vi "ACal-Create Cal Sweep.vi"(8 "error in (no error)":errorcluster, 11 "Cal Stimulus":T1={"Min Freq (Hz)"=50.0, "Max Freq (Hz)"=50000.0, "Freq Step (Hz)"=50.0, "Waveform"=enum."Chirp", "Attenuation (dB)"=20.0, "Sample Rate (Hz)"=100000.0}) -> (0 "error out":errorcluster, 2 "Stimulus waveform":cluster{i32, dbl, dbl[]}, 3 "Stimulus":dbl[](array[numeric]))   [LabVIEW 2020]
uses:
  Type Defs/Cal Stimulus.ctl
  <vilib>/Analysis/2dsp.llb/Inverse Complex FFT.vi
  <vilib>/Analysis/NI_AALPro.lvlib
panel:
  out "Phase graph":cluster{i32, "Freq Step (Hz)":dbl, dbl[]}(graph)
  out "Magnitude graph":cluster{i32, "Freq Step (Hz)":dbl, dbl[]}(graph)
  out "Signal graph":cluster{i32, dbl, dbl[]}(graph)
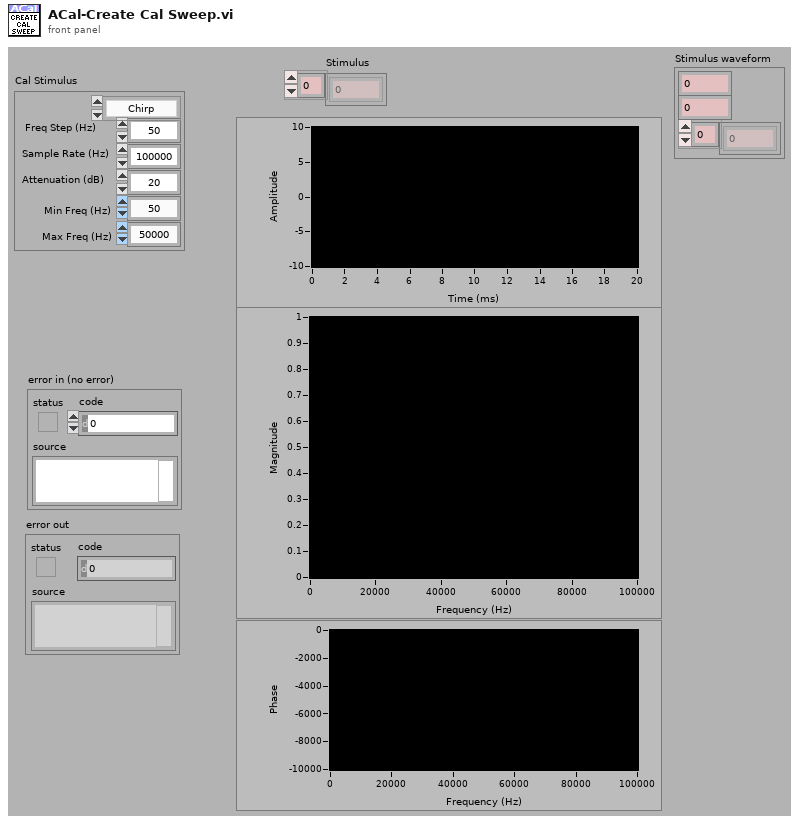
[diagram p1: front panel]
types:
  T1 = typedef "Cal Stimulus.ctl" = cluster{"Min Freq (Hz)":dbl, "Max Freq (Hz)":dbl, "Freq Step (Hz)":dbl, "Waveform":enum16{"Chirp", "Weighted"}, "Attenuation (dB)":dbl, "Sample Rate (Hz)":dbl}
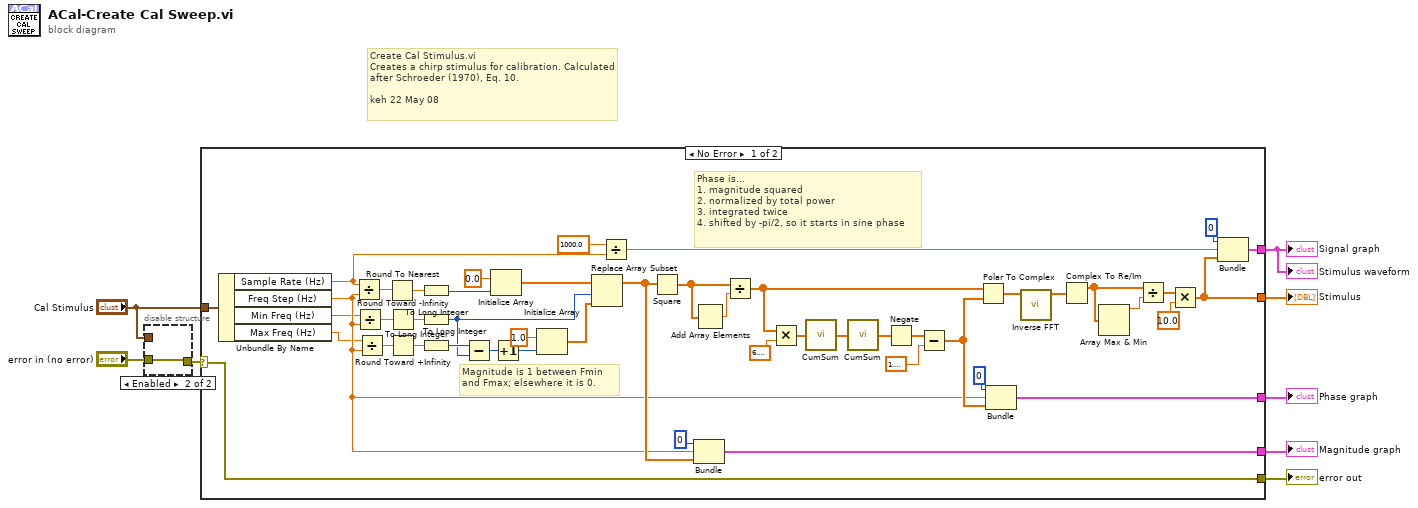
[diagram p0: block diagram]
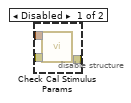
[diagram p2: hidden frame]
diagram:
  # "Create Cal Stimulus.vi\nCreates a chirp stimulus for calibration. Calculated after Schroeder (1970), Eq. 10.\n\nkeh 22 May 08"
  n1 = disable-structure shown="Enabled" {
    disable-tunnel: "Cal Stimulus" -> [w11 _]
    disable-tunnel: [w10 w12] -> w4
    disable-tunnel: "error in (no error)" -> [w9 w12]
    frame Disabled {
      n2 = call "Check Cal Stimulus Params.vi"("error in (no error)"=w9, "Cal Stimulus"=w11) -> ("error out"=w10:errorcluster)  [unwired: 9 in]
    }
    frame Enabled {
    }
  }
  n3 = case shown="No Error" w4 {
    selector: w4 -> [w20 w60]
    tunnel: "Cal Stimulus" -> [w59 _]
    tunnel: [w58 _] -> w8
    tunnel: [w57 _] -> w7
    tunnel: [w56 _] -> w6
    tunnel: [w55 _] -> w1
    tunnel: [w20 w60] -> w2
    frame No Error {
      # "Phase is...\n1. magnitude squared\n2. normalized by total power\n3. integrated twice\n4. shifted by -pi/2, so it starts in sine phase"
      # "Magnitude is 1 between Fmin\nand Fmax; elsewhere it is 0."
      n4 = Unbundle By Name(w59) -> ("Sample Rate (Hz)"=w16:dbl, "Freq Step (Hz)"=w15:dbl, "Min Freq (Hz)"=w14:dbl, "Max Freq (Hz)"=w13:dbl)
      n5 = Divide(x=w16, y=w15) -> (x/y=w54:dbl)
      n6 = Divide(x=w14, y=w15) -> (x/y=w50:dbl)
      n7 = Divide(x=w13, y=w15) -> (x/y=w49:dbl)
      n8 = Round To Nearest(number=w54) -> (nearest integer value=w53:dbl)
      n9 = Round Toward -Infinity(1:w50) -> (0:w47:dbl)
      n10 = Round Toward +Infinity(x=w49) -> (ceil(x): smallest int >= x=w48:dbl)
      n11 = To Long Integer(number=w53) -> (32bit integer=w52:i32)
      n12 = To Long Integer(number=w47) -> (32bit integer=w43:i32)
      n13 = To Long Integer(number=w48) -> (32bit integer=w44:i32)
      n14 = Subtract(x=w44, y=w43) -> (x-y=w42:i32)
      n15 = Initialize Array(0.0 ("element"), w52) -> (w46:dbl[])
      n16 = Increment(x=w42) -> (x+1=w41:i32)
      n17 = Initialize Array(1.0 ("element"), w41) -> (w40:dbl[])
      n18 = Replace Array Subset(array=w46, new element=w40, index=w43) -> (w38:dbl[])
      n19 = Divide(x=1000.0, y=w16) -> (x/y=w22:dbl)
      n20 = Square(x=w38) -> (x^2=w37:dbl[])
      n21 = Bundle(0, "Freq Step (Hz)"=w15, w38) -> (w58:cluster{i32, "Freq Step (Hz)":dbl, dbl[]})  [unwired: 1 in]
      n22 = Add Array Elements(numeric array=w37) -> (sum=w36:dbl)
      n23 = Divide(x=w37, y=w36) -> (x/y=w30:dbl[])
      n24 = Multiply(x=w30, y=6.283185307179586) -> (x*y=w34:dbl[])
      n25 = call "CumSum.vi"("Array"=w34) -> ("CumSum"=w33:dbl[])
      n26 = call "CumSum.vi"("Array"=w33) -> ("CumSum"=w32:dbl[])
      n27 = Negate(x=w32) -> (-x=w27:dbl[])
      n28 = Subtract(x=w27, y=1.5707963267948966) -> (x-y=w26:dbl[])
      n29 = Polar To Complex(1:w26, 2:w30) -> (0:w29:cdb[])
      n30 = Bundle(0, "Freq Step (Hz)"=w15, w26) -> (w57:cluster{i32, "Freq Step (Hz)":dbl, dbl[]})  [unwired: 1 in]
      n31 = call-poly <vilib>:"Inverse FFT.vi"("FFT {X}"=w29) -> ("X"=w28:cdb[])  [unwired: 9 in, 1 out]
      n32 = Complex To Re/Im(x + iy=w28) -> (x=w21:dbl[])  [unwired: 1 out]
      n33 = Array Max & Min(array=w21) -> (max value=w19:dbl)  [unwired: 3 out]
      n34 = Divide(x=w21, y=w19) -> (x/y=w18:dbl[])
      n35 = Multiply(x=w18, y=10.0) -> (x*y=w55:dbl[])
      n36 = Bundle(0, w22, w55) -> (w56:cluster{i32, dbl, dbl[]})  [unwired: 1 in]
    }
    frame Error {
    }
  }
  "Stimulus" <- w1
  "Signal graph" <- w6
  "Magnitude graph" <- w8
  "Phase graph" <- w7
  "Stimulus waveform" <- w6
  "error out" <- w2
